vi "Register Suite.vi"(11 "Properties.Suite in":refnum<class "Properties.Suite.lvclass">) -> (3 "Properties.Suite out":refnum<class "Properties.Suite.lvclass">)   [LabVIEW 2013, in "Caraya.lvlib" / "Properties.Suite.lvclass"]
uses:
  Properties.Suite.lvclass
  Test Manager Message Test/Test-Data -- cluster.ctl
  Properties/Properties.lvclass/Properties.ctl
  Properties/Properties.lvclass
  Test Manager Message Test/TestManagerMsg.Test.lvclass
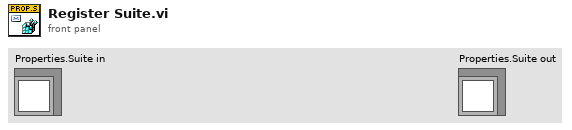
[diagram p1: front panel]
types:
  T1 = typedef "Caraya.lvlib/TestManagerMsg.Test.lvclass/Test-Data -- cluster.ctl" = cluster{"test-name":string, "call-chain":string[], "timestamp":timestamp}
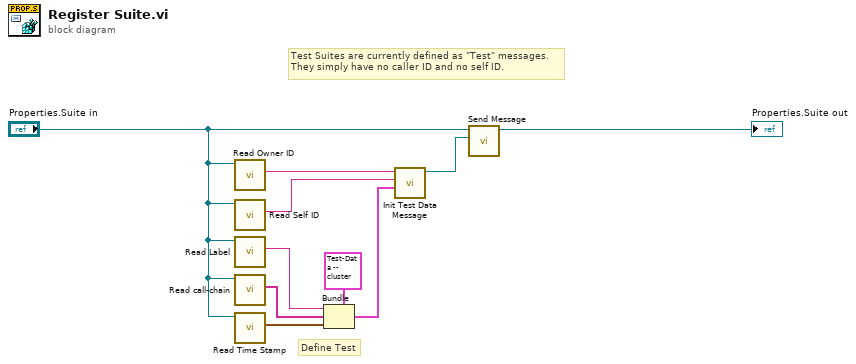
[diagram p0: block diagram]
diagram:
  # "Test Suites are currently defined as \"Test\" messages.\nThey simply have no caller ID and no self ID."
  # "Define Test"
  n1 = call "Read Owner ID.vi"("Properties in"="Properties.Suite in") -> ("owner-id"=w3:string)  [unwired: 9 in, 1 out]
  n2 = call "Read Self ID.vi"("Properties in"="Properties.Suite in") -> ("self-id"=w4:string)  [unwired: 9 in, 1 out]
  n3 = call "Read Label.vi"("Properties in"="Properties.Suite in") -> ("Test Label"=w7:string)  [unwired: 9 in, 1 out]
  n4 = call "Read call-chain.vi"("Properties in"="Properties.Suite in") -> ("call-chain"=w9:string[])  [unwired: 9 in, 1 out]
  n5 = call "Read Time Stamp.vi"("Properties in"="Properties.Suite in") -> ("Time Stamp"=w8:timestamp)  [unwired: 9 in, 1 out]
  n6 = Bundle(cluster=T1 {"test-name"="", "call-chain"=[], "timestamp"=timestamp(3763321070.9484735 s since 1904-01-01)} ("Test Data"), "test-name"=w7, "call-chain"=w9, "timestamp"=w8) -> (w5:T1)
  n7 = call "Init Test Data Message.vi"("Test Data"=w5, "TestID"=w4, "CallerID"=w3) -> ("Message"=w10:refnum<class "TestManagerMsg.lvclass">)  [unwired: 8 in]
  n8 = call "Send Message.vi"("TestManagerMsg"=w10, "Properties in"="Properties.Suite in") -> ("Properties out"=→"Properties.Suite out":refnum<class "Properties.Suite.lvclass">)  [unwired: 8 in, 1 out]
